vi "SendSETAndWaitForACK.vi"(0 "connection ID":refnum<k5>, 1 "Signature":u32, 2 "Active SET":string, 4 "Value (little endianed byte array)":u8[](array[numeric]), 5 "Error IN":errorcluster, 9 "path_config":path=path "C:/BonOMM/BonOMM 7.1/BonOMM 7.1.vi" caption="Command.ini") -> (14 "connection ID (dup)":refnum<k5>, 19 "Error OUT":errorcluster)   [LabVIEW 2019]
panel:
  out "CommandEnum":string[](array[string])
  out "TypeEnum":u32[](array[numeric])
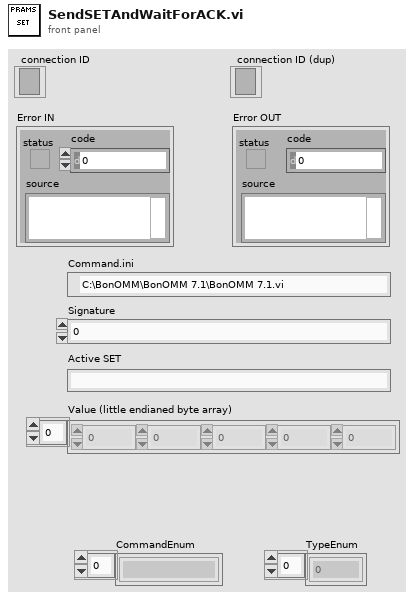
[diagram p1: front panel]
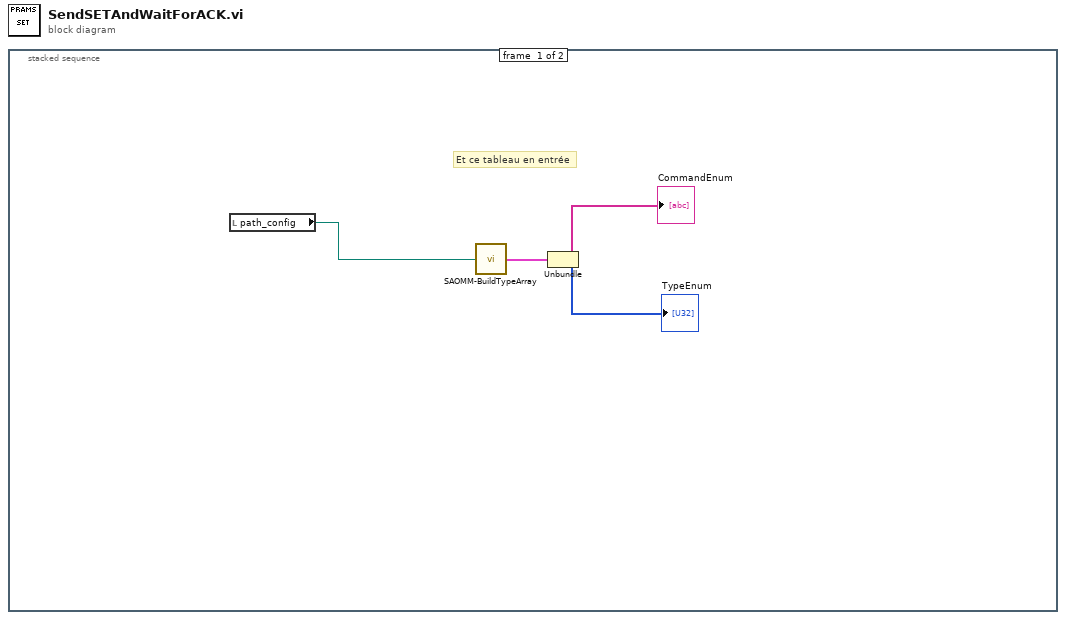
[diagram p0: block diagram]
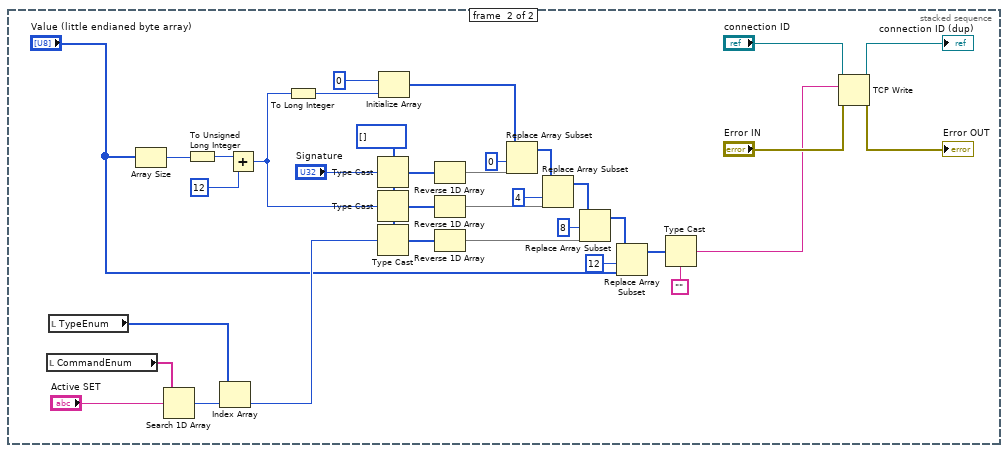
[diagram p2: hidden frame]
diagram:
  n1 = stacked-sequence {
    frame #0 {
      # "Et ce tableau en entrée"
      n2 = local read "path_config"() -> (w1:path)
      n3 = call "SAOMM-BuildTypeArray.vi"("command.ini"=w1) -> ("CommandArray"=w4:cluster{string[], u32[]})  [unwired: 14 in]
      n4 = Unbundle(w4) -> (→"CommandEnum":string[], →"TypeEnum":u32[])
    }
    frame #1 {
      w38 = u8[] []
      n5 = local read "CommandEnum"() -> (w28:string[])
      n6 = local read "TypeEnum"() -> (w26:u32[])
      n7 = Array Size(array="Value (little endianed byte array)") -> (size(s)=w39:i32)
      n8 = Search 1D Array(1D array=w28, element="Active SET") -> (index of element=w27:i32)  [unwired: 1 in]
      n9 = To Unsigned Long Integer(number=w39) -> (unsigned 32bit integer=w6:u32)
      n10 = Index Array(array=w26, index=w27) -> (element=w25:u32)
      n11 = Add(x=w6, y=u32 12 ("x")) -> (x+y=w23:u32)
      n12 = To Long Integer(number=w23) -> (32bit integer=w22:i32)
      n13 = Type Cast(type=w38, x="Signature") -> (*(type *) &x=w35:u8[])
      n14 = Type Cast(type=w38, x=w23) -> (*(type *) &x=w37:u8[])
      n15 = Type Cast(type=w38, x=w25) -> (*(type *) &x=w36:u8[])
      n16 = Initialize Array(u8 0, w22) -> (w14:u8[])
      n17 = Reverse 1D Array(array=w35) -> (reversed array=w10:u8[])
      n18 = Reverse 1D Array(array=w37) -> (reversed array=w9:u8[])
      n19 = Reverse 1D Array(array=w36) -> (reversed array=w8:u8[])
      n20 = Replace Array Subset(array=w14, new element=w10, index=0) -> (w21:u8[])
      n21 = Replace Array Subset(array=w21, new element=w9, index=4) -> (w20:u8[])
      n22 = Replace Array Subset(array=w20, new element=w8, index=8) -> (w19:u8[])
      n23 = Replace Array Subset(array=w19, new element="Value (little endianed byte array)", index=12) -> (w13:u8[])
      n24 = Type Cast(type="", x=w13) -> (*(type *) &x=w11:string)
      n25 = TCP Write(connection ID="connection ID", data in=w11, error in (no error)="Error IN") -> (connection ID out=→"connection ID (dup)":refnum<k5>, error out=→"Error OUT":errorcluster)  [unwired: 1 in, 1 out]
    }
  }
